vi "Calculate Gamma.vi"(4 "Port (Port 1)":u16(ring) items=["Port 1", "Port 2"], 5 "Termination":cdb[](array[numeric]), 6 "error in (no error)":errorcluster, 9 "2-port S-parameters":cdb[][](array[numeric])) -> (0 "error out":errorcluster, 3 "Gamma":cdb[](array[numeric]))   [LabVIEW 2023, in "NI_HFNetworkAnalysis.lvlib"]
doc: "Calculates the reflection factor, for different frequencies, at the specified port of a 2-port network while the other port is terminated with the specified termination. \n\nThe network is described by 2-port S-parameters <b>(S11,S12,S21,S22)</b> at different frequencies and the termination is described by its reflection factor at those frequencies.\n\n<b>Known Limitations</b>\nOnly 2-port networks are supported."
uses:
  NI_HFNetworkAnalysis.lvlib
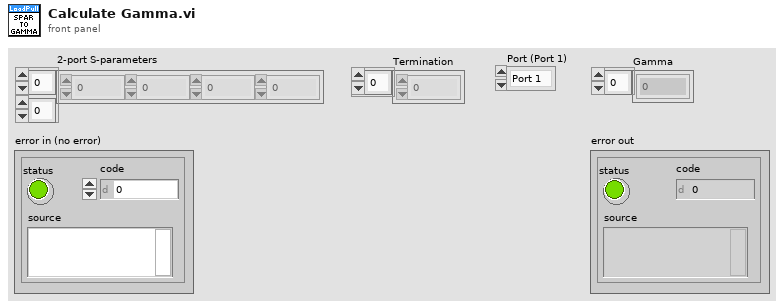
[diagram p1: front panel]
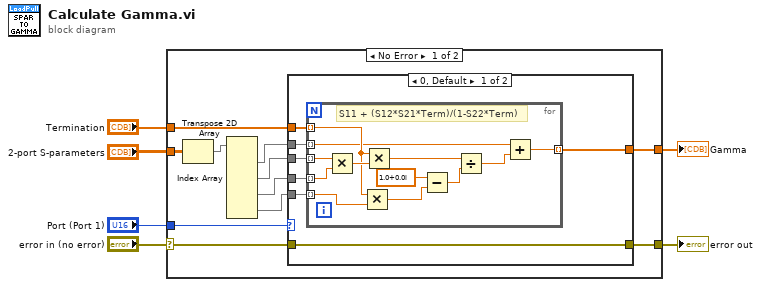
[diagram p0: block diagram]
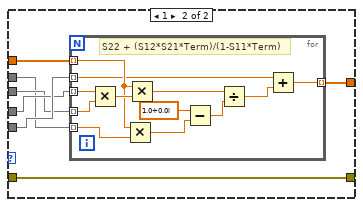
[diagram p2: hidden frame]
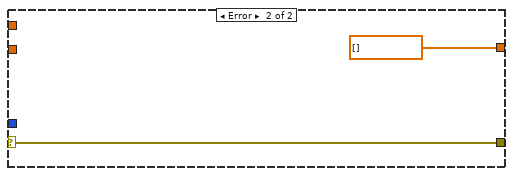
[diagram p3: hidden frame]
diagram:
  n1 = case shown="No Error" "error in (no error)" {
    selector: "error in (no error)" -> [w9 w57]
    tunnel: "Termination" -> [w17 _]
    tunnel: [w16 cdb[] []] -> w5
    tunnel: "2-port S-parameters" -> [w15 _]
    tunnel: "Port (Port 1)" -> [w11 _]
    tunnel: [w10 w57] -> w2
    frame No Error {
      n2 = Transpose 2D Array(2D array=w15) -> (transposed array=w14:cdb[][])
      n3 = Index Array(array=w14) -> (element #1=w13:cdb[], element #2=w8:cdb[], element #3=w7:cdb[], element #4=w12:cdb[])  [unwired: 8 in]
      n4 = case shown="0, Default" w11 {
        tunnel: w17 -> [w24 w43]
        tunnel: [w23 w38] -> w16
        tunnel: w13 -> [w22 w37]
        tunnel: w7 -> [w21 w41]
        tunnel: w8 -> [w20 w40]
        tunnel: w12 -> [w19 w42]
        tunnel: [w18 w39] -> w10
        tunnel: w9 -> [w18 w39]
        frame 0, Default {
          n5 = for {
            tunnel: w22 -> [w27] mode=indexing
            tunnel: w20 -> [w36] mode=indexing
            tunnel: w21 -> [w35] mode=indexing
            tunnel: w19 -> [w32] mode=indexing
            tunnel: w24 -> [w31] mode=indexing
            tunnel: [w25] -> w23 mode=indexing
            # "S11 + (S12*S21*Term)/(1-S22*Term)"
            n6 = Multiply(x=w36, y=w35) -> (x*y=w33:cdb)
            n7 = Multiply(x=w31, y=w32) -> (x*y=w30:cdb)
            n8 = Multiply(x=w31, y=w33) -> (x*y=w28:cdb)
            n9 = Subtract(x=cdb 1.0+0.0i, y=w30) -> (x-y=w29:cdb)
            n10 = Divide(x=w28, y=w29) -> (x/y=w26:cdb)
            n11 = Add(x=w27, y=w26) -> (x+y=w25:cdb)
          }
        }
        frame 1 {
          n12 = for {
            tunnel: w42 -> [w46] mode=indexing
            tunnel: w41 -> [w55] mode=indexing
            tunnel: w40 -> [w54] mode=indexing
            tunnel: w37 -> [w51] mode=indexing
            tunnel: w43 -> [w50] mode=indexing
            tunnel: [w44] -> w38 mode=indexing
            # "S22 + (S12*S21*Term)/(1-S11*Term)"
            n13 = Multiply(x=w55, y=w54) -> (x*y=w52:cdb)
            n14 = Multiply(x=w50, y=w51) -> (x*y=w49:cdb)
            n15 = Multiply(x=w50, y=w52) -> (x*y=w47:cdb)
            n16 = Subtract(x=cdb 1.0+0.0i, y=w49) -> (x-y=w48:cdb)
            n17 = Divide(x=w47, y=w48) -> (x/y=w45:cdb)
            n18 = Add(x=w46, y=w45) -> (x+y=w44:cdb)
          }
        }
      }
    }
    frame Error {
    }
  }
  "Gamma" <- w5
  "error out" <- w2
